vi "Sort_F_of_X.vi"(0 "F(x) - Evaluation Results":dbl[](array[numeric]), 2 "Sort Direction":enum16{"Low to High", "High to Low"}(ring), 11 "x Values - Amount of Modes":dbl[][](array[numeric])) -> (4 "Sorted F(x)":dbl[](array[numeric]), 15 "Sorted X Values":dbl[][](array[numeric]))   [LabVIEW 2014]
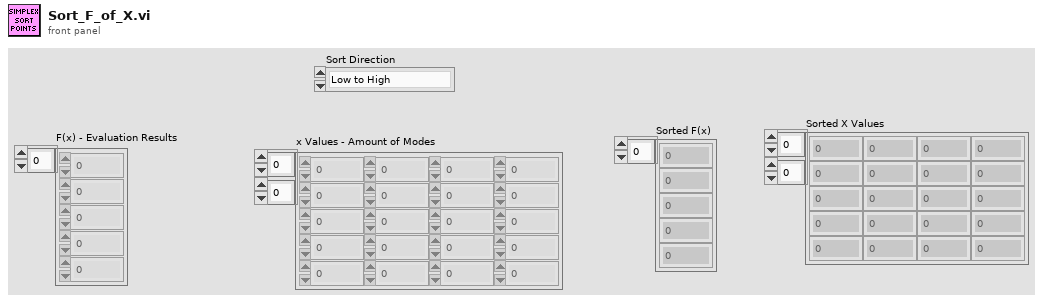
[diagram p1: front panel]
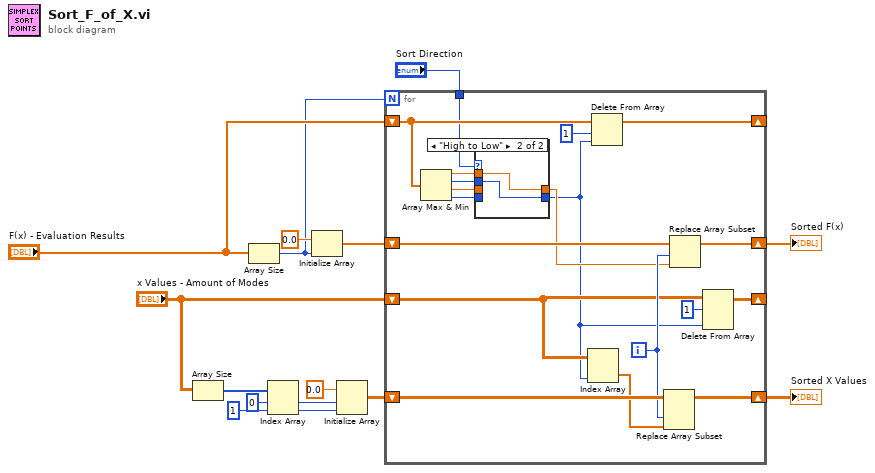
[diagram p0: block diagram]
diagram:
  n1 = Array Size(array="x Values - Amount of Modes") -> (size(s)=w5:i32[])
  n2 = Array Size(array="F(x) - Evaluation Results") -> (size(s)=w10:i32)
  n3 = Index Array(array=w5, index #1=0 ("index"), index #2=1 ("index")) -> (element #1=w2:i32, element #2=w1:i32)
  n4 = Initialize Array(0.0 ("element"), w10) -> (w12:dbl[])
  n5 = Initialize Array(0.0 ("element"), w2, w1) -> (w13:dbl[][])
  n6 = for {
    N: w10 -> [_]
    shift-right: [w26] -> w9
    shift-left: w12 -> [w34]
    shift-right: [w32] -> w8
    shift-left: w13 -> [w33]
    shift-right: [w30] -> _
    shift-left: "F(x) - Evaluation Results" -> [w31]
    shift-right: [w24] -> _
    shift-left: "x Values - Amount of Modes" -> [w25]
    tunnel: "Sort Direction" -> [w18]
    i -> [w28]
    n7 = Array Max & Min(array=w31) -> (max value=w17:dbl, max index (indices)=w16:i32, min value=w21:dbl, min index (indices)=w20:i32)
    n8 = case shown="\"High to Low\"" w18 {
      tunnel: w21 -> [w36 _]
      tunnel: [w36 w37] -> w22
      tunnel: w20 -> [w35 _]
      tunnel: [w35 w38] -> w19
      tunnel: w17 -> [_ w37]
      tunnel: w16 -> [_ w38]
      frame "Low to High", Default {
      }
      frame "High to Low" {
      }
    }
    n9 = Index Array(array=w25, index (col)=w19) -> (element=w27:dbl[])  [unwired: 1 in]
    n10 = Delete From Array(array=w31, length=1, index=w19) -> (array with subset deleted=w30:dbl[])  [unwired: 1 out]
    n11 = Replace Array Subset(array=w33, new element=w27, index (col)=w28) -> (w32:dbl[][])  [unwired: 1 in]
    n12 = Replace Array Subset(array=w34, new element=w22, index=w28) -> (w26:dbl[])
    n13 = Delete From Array(array=w25, length=1, index (col)=w19) -> (array with subset deleted=w24:dbl[][])  [unwired: 1 in, 1 out]
  }
  "Sorted F(x)" <- w9
  "Sorted X Values" <- w8
